vi "Read Device Identification.vi"(8 "error in (no error)":errorcluster, 9 "read device ID code":T1, 10 "object ID":u8, 11 "Modbus master in":refnum<class "Modbus Master.lvclass">) -> (0 "error out":errorcluster, 2 "objects":cluster{"object ID":u8, "value":string}[](array[cluster]) {"object ID" format="%x"}, 3 "Modbus master out":refnum<class "Modbus Master.lvclass">)   [LabVIEW 2021, in "Modbus Master.lvclass"]
doc: "Returns the device identification of a Modbus slave. Device identification consists of data elements called objects. Each object has an identification number and stores Modbus slave information."
uses:
  Modbus Master.lvclass
  Master Function Definition/Read Device ID code.ctl
  Modbus Master.lvclass/Modbus Master.ctl
  Modbus Data Unit/Modbus Data Unit.lvclass/Modbus Data Unit.ctl
  Network Protocol/Network Master/Network Master.lvclass/Network Master.ctl
  Master Function Definition/Read Device ID Type Request.vi
  Network Protocol/Network Master/Read write Master.vi
  Master Function Definition/Read Device Identification Response.vi
  Modbus Data Unit/Construct PDU.vi
  Master Function Definition/Convert to String.vi
  Master Function Definition/Function code mismatch error.vi
  Data Model/Error Generator.vi
  Modbus Data Unit/Deconstruct PDU.vi
  Modbus Data Unit/Modbus Data Unit.lvclass
  Transmission Data Unit/Transmission Data Unit.lvclass
  Network Protocol/Network Master/Network Master.lvclass
  Data Model/Device Data Model.lvclass
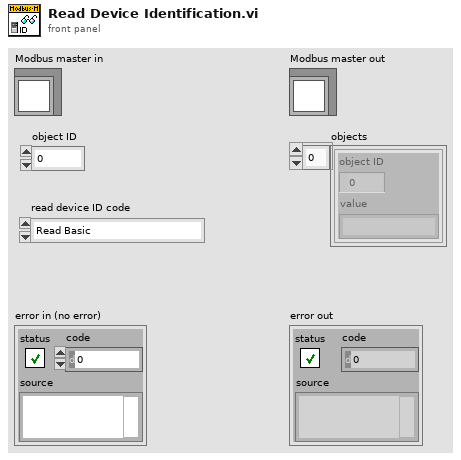
[diagram p1: front panel]
types:
  T1 = typedef "Device Data Model.lvclass/Read Device ID code.ctl" = enum8{"Read Basic", "Read Regular", "Read Extended", "Read Specific"}
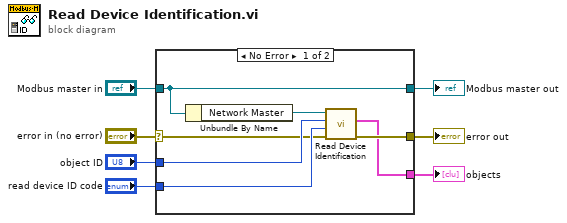
[diagram p0: block diagram]
diagram:
  n1 = case shown="No Error" "error in (no error)" {
    selector: "error in (no error)" -> [w9 w16]
    tunnel: "Modbus master in" -> [w8 w15]
    tunnel: [w8 w15] -> w5
    tunnel: [w14 w16] -> w4
    tunnel: "read device ID code" -> [w11 _]
    tunnel: "object ID" -> [w12 _]
    tunnel: [w13 _] -> w2
    frame No Error {
      n2 = Unbundle By Name(w8) -> ("Network Master"=w10:refnum<class "Network Master.lvclass">)
      n3 = call "Read Device Identification.vi"("error in (no error)"=w9, "read device ID code"=w11, "object ID"=w12, "Modbus master in"=w10) -> ("error out"=w14:errorcluster, "objects"=w13:cluster{"object ID":u8, "value":string}[])  [unwired: 5 in, 1 out]
    }
    frame Error {
    }
  }
  "error out" <- w4
  "Modbus master out" <- w5
  "objects" <- w2
